vi "Can Detection.vi"(9 "Stop Voltage":dbl, 10 "Direction (0-359)":dbl, 11 "Speed":dbl) -> (1 "Distance Reached?":bool, 2 "Joy Y":dbl=0.5124433303800191, 3 "Joy X":dbl)   [LabVIEW 2014]
uses:
  Begin/Global RefNums.vi
panel:
  out "Voltage":dbl
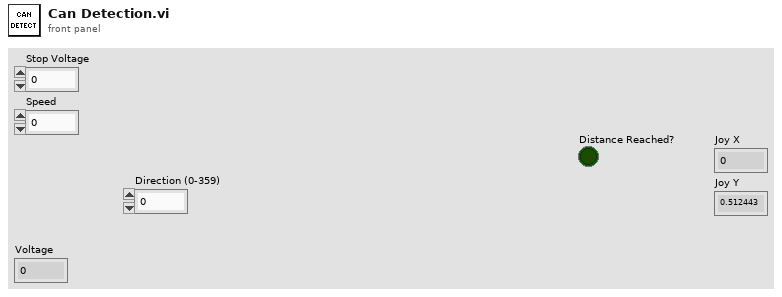
[diagram p1: front panel]
types:
  T1 = typedef "WPI_AnalogChannelDevRef.ctl" = cluster{"DevStatus":errorcluster, "Controller":T2, "Analog Channel":T3}
  T2 = typedef "FPGA_TypedefAnalogModule.ctl" = enum16{"Controller 1"}
  T3 = typedef "FPGA_AIChannel.ctl" = enum8{"AI 0", "AI 1", "AI 2", "AI 3", "AI MXP 0", "AI MXP 1", "AI MXP 2", "AI MXP 3", "Invalid"}
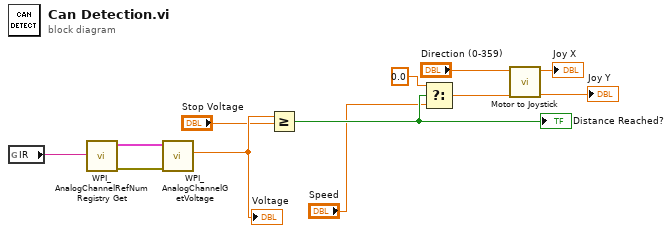
[diagram p0: block diagram]
diagram:
  n1 = global read "Global RefNums.vi" "IR"() -> (w7:string)
  n2 = call <vilib>:"WPI_AnalogChannelRefNum Registry Get.vi"("refnum name"=w7) -> ("error out"=w5:errorcluster, "AIDeviceRef"=w6:T1)  [unwired: 9 in]
  n3 = call <vilib>:"WPI_AnalogChannelGetVoltage.vi"("error in (no error)"=w5, "AIDeviceRef"=w6) -> ("Voltage"=w3:dbl)  [unwired: 7 in, 2 out]
  "Voltage" <- w3
  n4 = Greater Or Equal?(x=w3, y="Stop Voltage") -> (x >= y?=w4:bool)
  "Distance Reached?" <- w4
  n5 = Select(t=0.0, s=w4, f="Speed") -> (s? t:f=w11:dbl)
  n6 = call "Motor to Joystick.vi"("Drive Motor"=w11, "Rotational Motor"="Direction (0-359)") -> ("Joy Y"=→"Joy Y":dbl, "Joy X"=→"Joy X":dbl)  [unwired: 8 in]
